vi "Read slave address.vi"(8 "error in (no error)":errorcluster caption="에러 입력(에러 없음)", 11 "I2C 입력":refnum<class "I2C.lvclass">) -> (0 "error out":errorcluster caption="에러 출력", 2 "slave address":u8 format="%02x", 3 "I2C 출력":refnum<class "I2C.lvclass">)   [LabVIEW 2020, in "I2C.lvclass"]
uses:
  I2C.lvclass
  I2C.lvclass/I2C.ctl
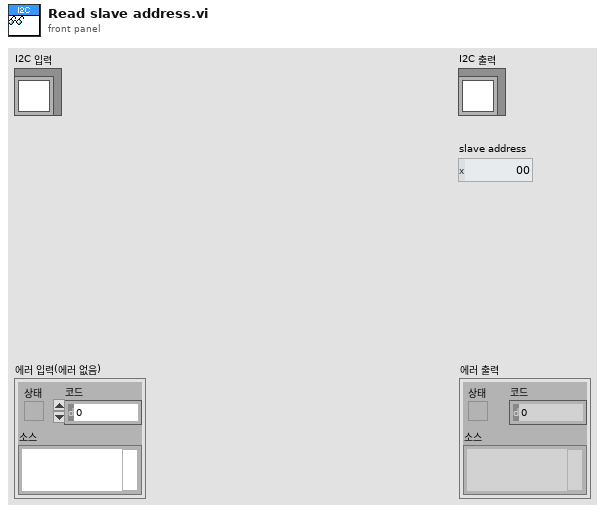
[diagram p1: front panel]
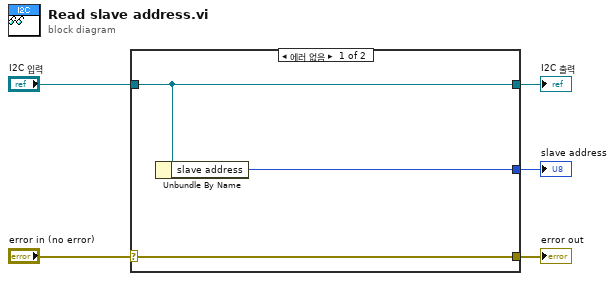
[diagram p0: block diagram]
diagram:
  n1 = case shown="에러 없음" "error in (no error)" {
    selector: "error in (no error)" -> [w8 w9]
    tunnel: [w8 w9] -> w4
    tunnel: [w7 w10] -> w2
    tunnel: "I2C 입력" -> [w7 w10]
    tunnel: [w6 _] -> w1
    frame No Error {
      n2 = Unbundle By Name(w7) -> ("slave address"=w6:u8)
    }
    frame Error {
    }
  }
  "error out" <- w4
  "I2C 출력" <- w2
  "slave address" <- w1
